vi "AI Configure.vi"(11 "settings in":T1 {"Simulated Signal"."amplitude" format="%.0pV"; "Simulated Signal"."frequency" format="%.2pHz"; "input range" format="%.0pV"; "sample rate" format="%.2pHz"}) -> ()   [LabVIEW 2019]
uses:
  subVIs/Measure and Log Settings.ctl
  subVIs/Simulated Signal Type.ctl
  <extravilib>/ChannelInstances/Tag-t'Measure and Log Settings.ctl'/Write With Abort.vi
  <extravilib>/ChannelInstances/Tag-t'Measure and Log Settings.ctl'/Endpoint.vi
  <extravilib>/ChannelInstances/Tag-t'Measure and Log Settings.ctl'.lvlib
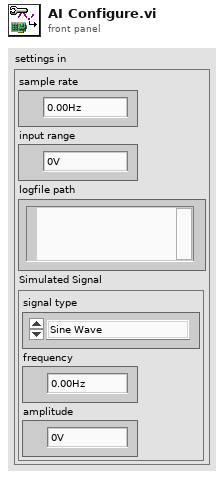
[diagram p1: front panel]
types:
  T1 = typedef "Measure and Log Settings.ctl" = cluster{"sample rate":dbl, "input range":dbl, "logfile path":path, "Simulated Signal":cluster{"signal type":T2, "frequency":dbl, "amplitude":dbl}}
  T2 = typedef "Simulated Signal Type.ctl" = enum16{"Sine Wave", "Square Wave with Noise"}
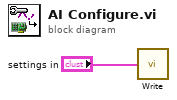
[diagram p0: block diagram]
diagram:
  n1 = call <extravilib>:"Write.vi"("element"="settings in") -> ()  [unwired: 2 out]
